vi "Read COM.vi"(8 "error in (no error)":errorcluster, 11 "Osciloscope in":refnum<class "Osciloscope.lvclass">) -> (0 "error out":errorcluster, 2 "COM":refnum<visa-resource-name>, 3 "Osciloscope out":refnum<class "Osciloscope.lvclass">)   [LabVIEW 2020, in "Osciloscope Tektronix.lvlib" / "Osciloscope.lvclass"]
uses:
  Osciloscope.lvclass
  Osciloscope.lvclass/Osciloscope.ctl
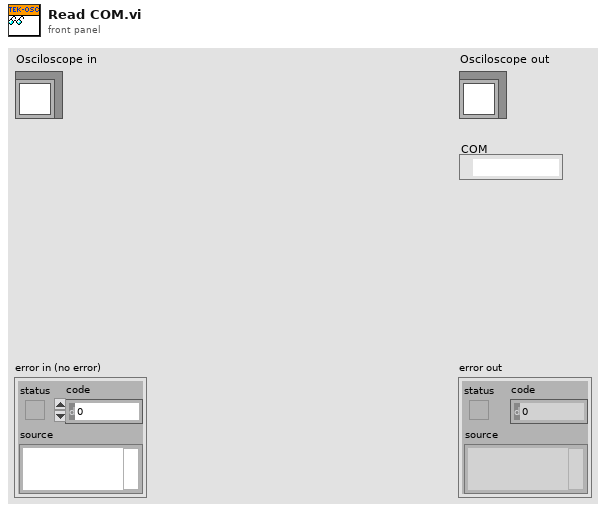
[diagram p1: front panel]
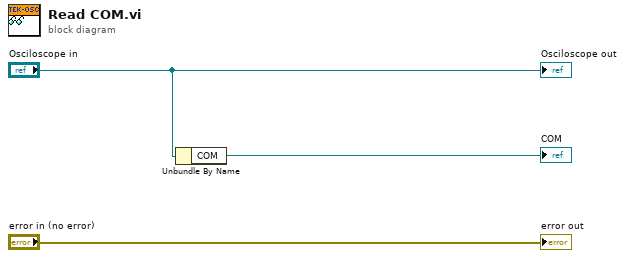
[diagram p0: block diagram]
diagram:
  n1 = Unbundle By Name("Osciloscope in") -> ("COM"=→"COM":refnum<visa-resource-name>)
  "error out" <- "error in (no error)"
  "Osciloscope out" <- "Osciloscope in"
